vi "finishPassToStrikerPlay.vi"(8 "error in (no error)":errorcluster, 10 "Game":refnum<class "Game.lvclass">, 11 "PassToStriker in":refnum<class "PassToStriker.lvclass">) -> (0 "error out":errorcluster, 2 "finishPassToStriker?":bool, 3 "PassToStriker out":refnum<class "PassToStriker.lvclass">)   [LabVIEW 2020, in "PassToStriker.lvclass"]
uses:
  PassToStriker.lvclass
  Game_class/Game.lvclass
  Referee_class/command_interpreted.ctl
  Utilities_class/Utilities.lvclass
  Game_class/Game.lvclass/Game.ctl
  Referee_class/Referee.lvclass/Referee.ctl
  Events_class/Events.lvclass/Events.ctl
  Object_class/Object.lvclass/Object.ctl
  Team_class/Team.lvclass/Team.ctl
  Game_class/Read EventsRef.vi
  Game_class/Read BallRef.vi
  Game_class/Read OffensiveTeam.vi
  Team_class/Read RobotRef.vi
  Object_class/Read x.vi
  Object_class/Read y.vi
  Events_class/Read touch.vi
  Events_class/Read id_touch.vi
  Events_class/Read ball_out.vi
  Game_class/Read Referee.vi
  Referee_class/Read command_interpreted.vi
  Ally_class/Ally.lvclass
  Ball_class/Ball.lvclass
  Referee_class/Referee.lvclass
  Events_class/Events.lvclass
  Robot_class/Robot.lvclass
  Play_class/Play.lvclass
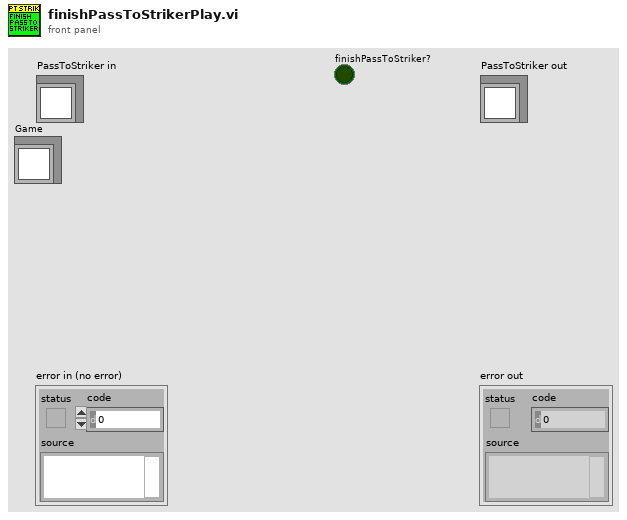
[diagram p1: front panel]
types:
  T1 = typedef "command_interpreted.ctl" = enum16{"Goal Ally", "Goal Enemy", "Ball Placement Enemy", "Ball Placement Ally", "Normal Half Time", "Extra Time  Break", "Extra Half Time", "None", "Post Game", "PKA Normal Start", "Prepare Kickoff Ally", "PKE Normal Start", "Prepare Kickoff Enemy", "Force Start", "Halt", "Timeout", "Prepare Penalty Ally", "Prepare Penalty Enemy", "PPA NormalStart", "PPE Normal Start", "Indirect Free Ally", "Direct Free Enemy", "Direct Free Ally", "Indirect Free Enemy", "Stop"}
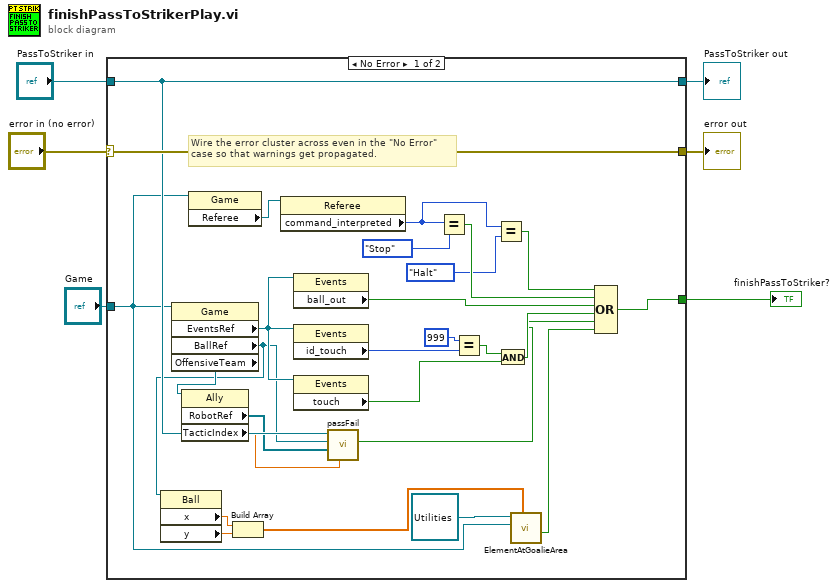
[diagram p0: block diagram]
diagram:
  n1 = case shown="No Error" "error in (no error)" {
    selector: "error in (no error)" -> [w33 w35]
    tunnel: [w33 w35] -> w5
    tunnel: [w18 w34] -> w3
    tunnel: "PassToStriker in" -> [w18 w34]
    tunnel: [w24 _] -> w2
    tunnel: "Game" -> [w8 _]
    frame No Error {
      # "Wire the error cluster across even in the \"No Error\"\ncase so that warnings get propagated."
      n2 = property class="Game"(reference=w8) -> ("EventsRef"=w32:refnum<class "Events.lvclass">, "BallRef"=w7:refnum<class "Ball.lvclass">, "OffensiveTeam"=w17:refnum<class "Ally.lvclass">)  [unwired: 1 in, 2 out]
      n3 = property class="Ball"(reference=w7) -> ("x"=w12:dbl, "y"=w11:dbl)  [unwired: 1 in, 2 out]
      n4 = property class="Ally"(reference=w17) -> ("RobotRef"=w16:refnum<class "Robot.lvclass">[], "TacticIndex"=w14:dbl)  [unwired: 1 in, 2 out]
      n5 = property class="Game"(reference=w8) -> ("Referee"=w26:refnum<class "Referee.lvclass">)  [unwired: 1 in, 2 out]
      n6 = Build Array(w12, w11) -> (w10:dbl[])
      n7 = property class="Referee"(reference=w26) -> ("command_interpreted"=w21:T1)  [unwired: 1 in, 2 out]
      n8 = property class="Events"(reference=w32) -> ("ball_out"=w29:bool)  [unwired: 1 in, 2 out]
      n9 = property class="Events"(reference=w32) -> ("id_touch"=w30:i32)  [unwired: 1 in, 2 out]
      n10 = property class="Events"(reference=w32) -> ("touch"=w25:bool)  [unwired: 1 in, 2 out]
      n11 = call "passFail.vi"("TacticIndex"=w14, "Offensive Robots"=w16, "Ball"=w7, "Play in"=w18) -> ("PassFail?"=w15:bool)  [unwired: 5 in, 2 out]
      n12 = Equal?(x=w21, y=command_interpreted."Stop") -> (x = y?=w22:bool)
      n13 = Equal?(x=999 ("id_touch"), y=w30) -> (x = y?=w28:bool)
      n14 = Equal?(x=w21, y=command_interpreted."Halt") -> (x = y?=w19:bool)
      n15 = And(x=w28, y=w25) -> (x .and. y?=w27:bool)
      n16 = call-dynamic "ElementAtGoalieArea.vi"("Elemento pos."=w10, "Game"=w8, "Utilities in"=refnum<class "Utilities.lvclass"> refnum) -> ("Element at ally goalkeeper area ?"=w9:bool)  [unwired: 5 in, 3 out]
      n17 = Compound Arithmetic op=OR(w19, w22, w29, w27, w15, w9) -> (w24:bool)
    }
    frame Error {
    }
  }
  "error out" <- w5
  "PassToStriker out" <- w3
  "finishPassToStriker?" <- w2
